vi "Pickup Floor.vi"(10 "Lift Height":dbl=3.0 format="%#_13g", 11 "Final Height":dbl format="%#_13g") -> ()   [LabVIEW 2014]
uses:
  Begin/Global Variables.vi
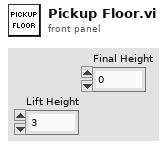
[diagram p1: front panel]
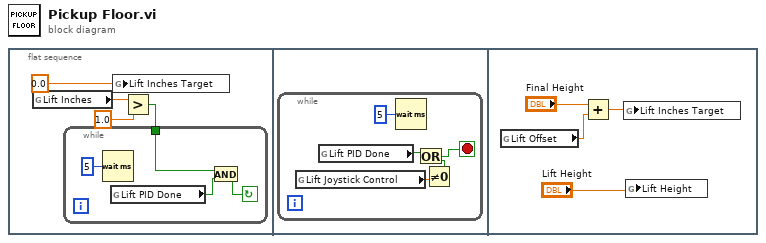
[diagram p0: block diagram]
diagram:
  n1 = flat-sequence {
    frame #0 {
      n2 = global read "Global Variables.vi" "Lift Inches"() -> (w2:dbl)
      n3 = global write "Global Variables.vi" "Lift Inches Target"(0.0 ("x")) -> ()
      n4 = Greater?(x=w2, y=1.0) -> (0:w1:bool)
      n5 = while {
        tunnel: w1 -> [w5]
        stop <- w6 continue-if-true
        n6 = Wait (ms)(milliseconds to wait=u32 5) -> ()  [unwired: 1 out]
        n7 = global read "Global Variables.vi" "Lift PID Done"() -> (w7:bool)
        n8 = And(x=w5, y=w7) -> (x .and. y?=w6:bool)
      }
    }
    frame #1 {
      n9 = while {
        stop <- w9 stop-if-true
        n10 = global read "Global Variables.vi" "Lift Joystick Control"() -> (w12:dbl)
        n11 = global read "Global Variables.vi" "Lift PID Done"() -> (w10:bool)
        n12 = Wait (ms)(milliseconds to wait=u32 5) -> ()  [unwired: 1 out]
        n13 = Not Equal To 0?(x=w12) -> (x != 0?=w11:bool)
        n14 = Or(x=w10, y=w11) -> (x .or. y?=w9:bool)
      }
    }
    frame #2 {
      n15 = global read "Global Variables.vi" "Lift Offset"() -> (w15:dbl)
      n16 = Add(x="Final Height", y=w15) -> (x+y=w17:dbl)
      n17 = global write "Global Variables.vi" "Lift Inches Target"(w17) -> ()
      n18 = global write "Global Variables.vi" "Lift Height"("Lift Height") -> ()
    }
  }
